vi "SRV_Check Product Name.vi"(3 "String":string) -> (1 "Not Valid":bool)   [LabVIEW 2015]
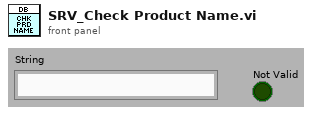
[diagram p1: front panel]
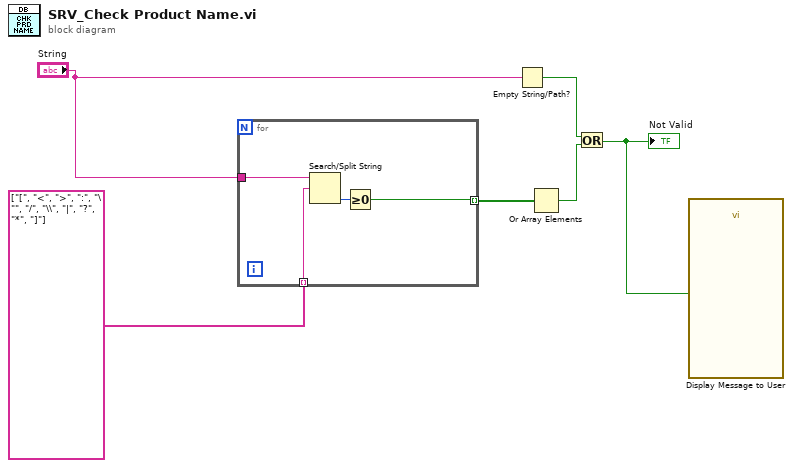
[diagram p0: block diagram]
diagram:
  n1 = for {
    tunnel: "String" -> [w9]
    tunnel: [w8] -> w6 mode=indexing
    tunnel: string[] ["[", "<", ">", ":", "\"", "/", "\\", "|", "?", "*", "]"] -> [w7] mode=indexing
    n2 = Search/Split String(string=w9, search string/char (-)=w7) -> (offset of match=w10:i32)  [unwired: 1 in, 2 out]
    n3 = Greater Or Equal To 0?(x=w10) -> (x >= 0?=w8:bool)
  }
  n4 = Empty String/Path?(string/path="String") -> (empty?=w3:bool)
  n5 = Or Array Elements(Boolean array=w6) -> (logical OR=w2:bool)
  n6 = Or(x=w3, y=w2) -> (x .or. y?=w1:bool)
  "Not Valid" <- w1
  n7 = call "Display Message to User"("Enable"=w1) -> ()  [unwired: 9 in, 2 out]
